vi "fgv_demo.vi"() -> ()   [LabVIEW 2021]
doc: "本VI是为《我和LabVIEW》一书编写的示例。\n关于本书的介绍请参考网页：\nhttp://ruanqizhen.spaces.live.com/blog/cns!5852D4F797C53FB6!4310.entry"
uses:
  fgv_function.ctl
panel:
  out "count 2":i32
  out "count":i32
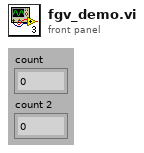
[diagram p1: front panel]
types:
  T1 = typedef "fgv_function.ctl" = enum16{"Reset", "Increase", "Decrease", "Read"}
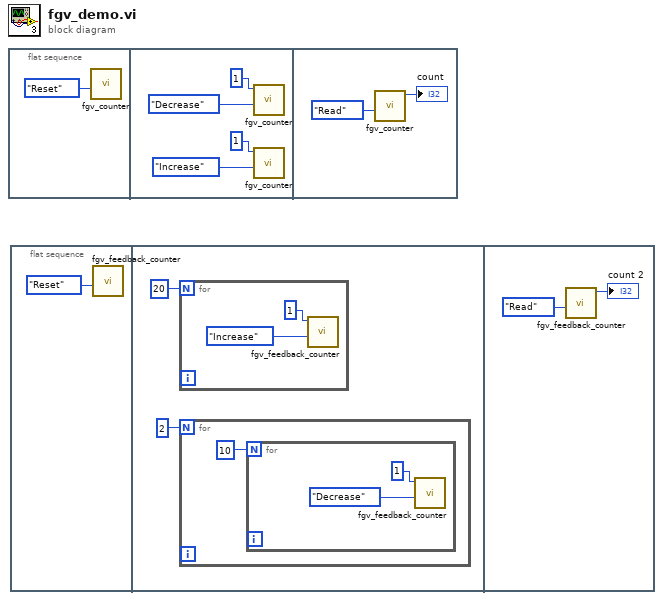
[diagram p0: block diagram]
diagram:
  n1 = flat-sequence {
    frame #0 {
      n2 = call "fgv_counter.vi"("function"=fgv_function."Reset") -> ()  [unwired: 10 in, 1 out]
    }
    frame #1 {
      n3 = call "fgv_counter.vi"("function"=fgv_function."Decrease", "data in"=1 ("数据输入")) -> ()  [unwired: 9 in, 1 out]
      n4 = call "fgv_counter.vi"("function"=fgv_function."Increase", "data in"=1 ("数据输入")) -> ()  [unwired: 9 in, 1 out]
    }
    frame #2 {
      n5 = call "fgv_counter.vi"("function"=fgv_function."Read") -> ("data out"=→"count":i32)  [unwired: 10 in]
    }
  }
  n6 = flat-sequence {
    frame #0 {
      n7 = call "fgv_feedback_counter.vi"("function"=fgv_function."Reset") -> ()  [unwired: 10 in, 1 out]
    }
    frame #1 {
      n8 = for {
        N: 20 -> [_]
        n9 = call "fgv_feedback_counter.vi"("function"=fgv_function."Increase", "data in"=1 ("数据输入")) -> ()  [unwired: 9 in, 1 out]
      }
      n10 = for {
        N: 2 -> [_]
        n11 = for {
          N: 10 -> [_]
          n12 = call "fgv_feedback_counter.vi"("function"=fgv_function."Decrease", "data in"=1 ("数据输入")) -> ()  [unwired: 9 in, 1 out]
        }
      }
    }
    frame #2 {
      n13 = call "fgv_feedback_counter.vi"("function"=fgv_function."Read") -> ("data out"=→"count 2":i32)  [unwired: 10 in]
    }
  }
